vi "ExBackAsyncExample.vi"() -> ()   [LabVIEW 2010]
panel:
  in  "Exposure":dbl format="%.2f"
  in  "stop":bool
  in  "Store":bool
  out "error out":errorcluster
  in  "error in (no error)":errorcluster
  # "ExBackAsyncExample:\nThis example  first takes a background file, then displays live data \nsubtracted by the first image taken until the stop button is hit."
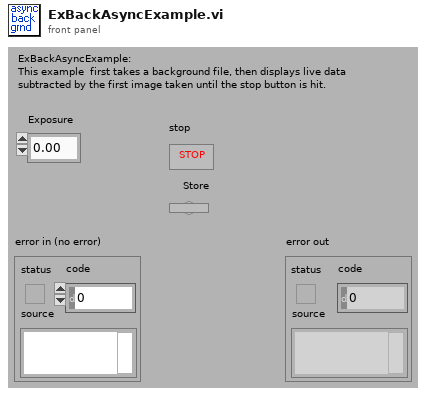
[diagram p1: front panel]
types:
  T1 = cluster{i32, "Xdim":u32, i32, i32, "Ydim":u32, i32}
  T2 = cluster{"Acquire mode (async)":i32, "Exposure":dbl, "Number of images":i32, "Software accumulation":i32}
  T3 = cluster{"Camera Handle":u32, "Pulser Handle":u32, "File Handle":u32, "Display Handle":u32, "Image Handle":u32}
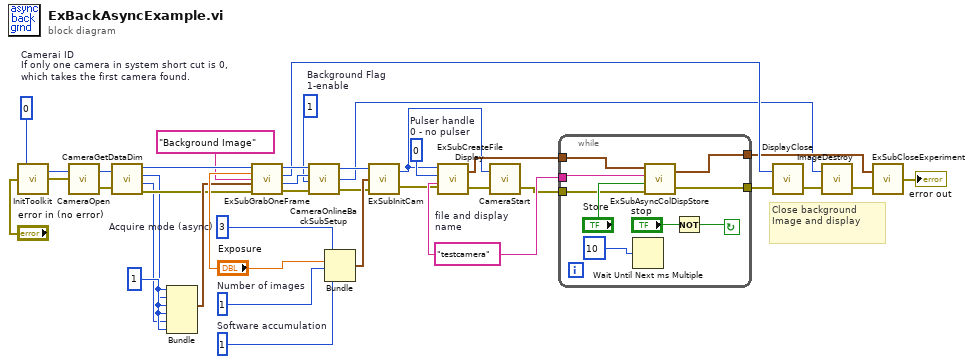
[diagram p0: block diagram]
diagram:
  w14 = 1
  w18 = 1  # Background Flag 1-enable
  w23 = 0  # Camerai ID If only one camera in system short cut is 0,  which takes the first camera found.
  w30 = 0  # Pulser handle 0 - no pulser
  w35 = 1  # Number of images
  w36 = 3  # Acquire mode (async)
  w34 = 1  # Software accumulation
  w37 = "testcamera"  # file and display name
  # "Close background\nImage and display"
  n1 = call <userlib>:"InitToolkit.vi"("error in"="error in (no error)") -> ("error out"=w24:errorcluster)
  n2 = call <userlib>:"CameraOpen.vi"("error in"=w24, "Camera Device ID"=w23) -> ("error out"=w12:errorcluster, "Camera Handle"=w16:u32)
  n3 = call <userlib>:"CameraGetDataDim.vi"("Camera Handle"=w16, "error in"=w12) -> ("Camera Handle"=w15:u32, "Xdim"=w2:u32, "Ydim"=w1:u32, "error out"=w11:errorcluster)
  n4 = Bundle(w14, "Xdim"=w2, w14, w14, "Ydim"=w1, w14) -> (w13:T1)  [unwired: 1 in]
  n5 = call "ExSubGrabOneFrame.vi"("Display Title"="Background Image", "error in"=w11, "ROI Cluster"=w13, "Exposure"="Exposure", "Camera Handle"=w15) -> ("error out"=w17:errorcluster, "Image Handle"=w19:u32, "Display Handle"=w9:u32, "Camera Handle out"=w20:u32)
  n6 = call <userlib>:"CameraOnlineBackSubSetup.vi"("error in"=w17, "Background Flag"=w18, "Background Image Handle"=w19, "Camera Handle"=w20) -> ("error out"=w21:errorcluster, "Background Image Handle"=w3:u32, "Camera Handle"=w22:u32)
  n7 = Bundle("Acquire mode (async)"=w36, "Exposure"="Exposure", "Number of images"=w35, "Software accumulation"=w34) -> (w32:T2)  [unwired: 1 in]
  n8 = call "ExSubInitCam.vi"("error in (no error)"=w21, "Camera Information"=w32, "Camera Handle"=w22) -> ("error out"=w31:errorcluster, "Camera Handle"=w26:u32)
  n9 = call "ExSubCreateFileDisplay.vi"("error in (no error)"=w31, "File and Display Name"=w37, "Pulser Handle"=w30, "Camera Handle"=w26) -> ("error out"=w29:errorcluster, "Handles Out"=w28:T3)
  n10 = call <userlib>:"CameraStart.vi"("error in"=w29, "Camera Handle"=w26) -> ("error out"=w27:errorcluster)  [unwired: 1 out]
  n11 = while {
    tunnel: w28 -> [w44]
    tunnel: w27 -> [w42]
    tunnel: w37 -> [w43]
    tunnel: [w40] -> w7
    tunnel: [w41] -> w6
    stop <- w39 continue-if-true
    n12 = Wait Until Next ms Multiple(millisecond multiple=10) -> ()  [unwired: 1 out]
    n13 = call "ExSubAsyncColDispStore.vi"("error in (no error)"=w42, "Store Data"="Store", "Display Title"=w43, "Handle Cluster"=w44) -> ("error out"=w40:errorcluster, "Handle Cluster Out"=w41:T3)
    n14 = Not(x="stop") -> (.not. x?=w39:bool)
  }
  n15 = call <userlib>:"DisplayClose.vi"("error in"=w7, "Display Handle"=w9) -> ("error out"=w8:errorcluster)
  n16 = call <userlib>:"ImageDestroy.vi"("error in"=w8, "Data handle"=w3) -> ("error out"=w5:errorcluster)
  n17 = call "ExSubCloseExperiment.vi"("error in (no error)"=w5, "Handles In"=w6) -> ("error out"=→"error out":errorcluster)
